vi "Move Main VI Controls.vi"(8 "error in":errorcluster, 11 "VIRef in":refnum<vi>) -> (0 "error out":errorcluster)   [LabVIEW 2018]
uses:
  <vilib>/Utility/miscctls.llb/LVPointTypeDef.ctl
panel:
  out "Height":i16
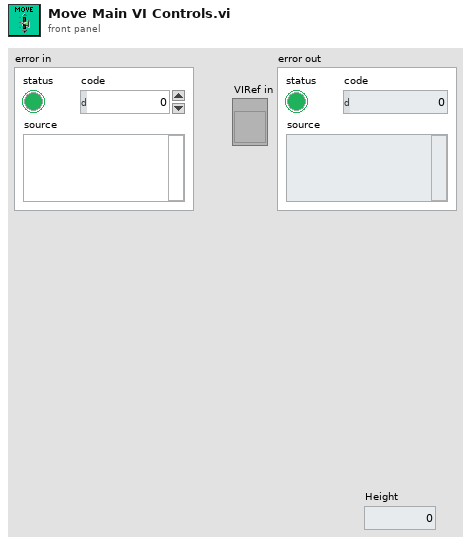
[diagram p1: front panel]
types:
  T1 = typedef "LVPointTypeDef.ctl" = cluster{"Horizontal":i16, "Vertical":i16}
  T2 = typedef "LVRectTypeDef.ctl" = cluster{"Left":i16, "Top":i16, "Right":i16, "Bottom":i16}
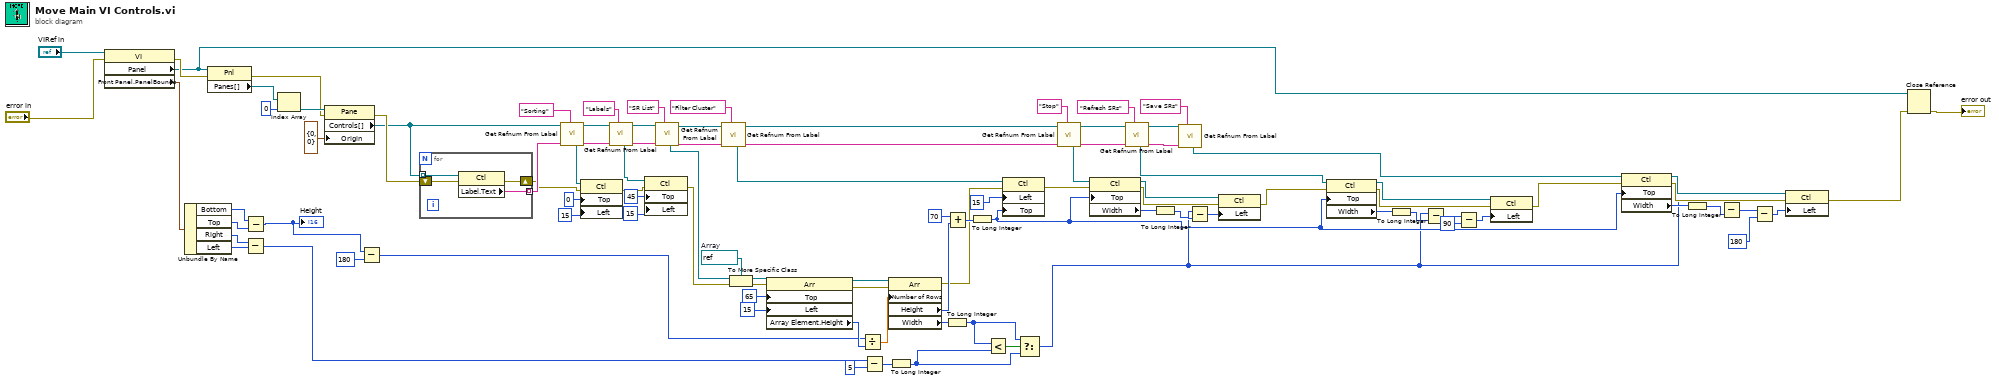
[diagram p0: block diagram]
diagram:
  w66 = refnum<vi> refnum  # Array
  n1 = property class="VI"(reference="VIRef in", error in="error in") -> (error out=w95:errorcluster, "Panel"=w3:refnum<vi>, "Front Panel.PanelBounds"=w92:T2)  [unwired: 1 out]
  n2 = Unbundle By Name(w92) -> ("Bottom"=w52:i16, "Top"=w51:i16, "Right"=w42:i16, "Left"=w41:i16)
  n3 = property class="Pnl"(reference=w3, error in=w95) -> (error out=w94:errorcluster, "Panes[]"=w96:refnum<vi>[])  [unwired: 1 out]
  n4 = Subtract(x=w42, y=w41) -> (x-y=w13:i16)
  n5 = Subtract(x=w52, y=w51) -> (x-y=w49:i16)
  "Height" <- w49
  n6 = Index Array(array=w96, index=0) -> (element=w97:refnum<vi>)
  n7 = property class="Pane"(reference=w97, error in=w94, "Origin"=T1 {"Horizontal"=0, "Vertical"=0}) -> (error out=w93:errorcluster, "Controls[]"=w90:refnum<vi>[])  [unwired: 1 out]
  n8 = Subtract(x=w49, y=i16 180) -> (x-y=w48:i16)
  n9 = for {
    tunnel: w90 -> [w102] mode=indexing
    shift-right: [w103] -> w58
    shift-left: w93 -> [w104]
    tunnel: [w101] -> w89 mode=indexing
    n10 = property class="Ctl"(reference=w102, error in=w104) -> (error out=w103:errorcluster, "Label.Text"=w101:string)  [unwired: 1 out]
  }
  n11 = call "Get Refnum From Label.vi"("label"="Sorting" ("element"), "label array in"=w89, "controls[] in"=w90) -> ("label array out"=w86:string[], "controls[] out"=w87:refnum<vi>[], "refnum out"=w70:refnum<vi>)  [unwired: 6 in]
  n12 = property class="Ctl"(reference=w70, error in=w58, "Top"=0 ("Position:Left"), "Left"=15 ("Position:Top")) -> (error out=w61:errorcluster)  [unwired: 1 out]
  n13 = call "Get Refnum From Label.vi"("label"="Labels" ("element"), "label array in"=w86, "controls[] in"=w87) -> ("label array out"=w83:string[], "controls[] out"=w84:refnum<vi>[], "refnum out"=w69:refnum<vi>)  [unwired: 6 in]
  n14 = property class="Ctl"(reference=w69, error in=w61, "Top"=45 ("Position:Top"), "Left"=15 ("Position:Left")) -> (error out=w60:errorcluster)  [unwired: 1 out]
  n15 = call "Get Refnum From Label.vi"("label"="SR List" ("element"), "label array in"=w83, "controls[] in"=w84) -> ("label array out"=w85:string[], "controls[] out"=w82:refnum<vi>[], "refnum out"=w67:refnum<vi>)  [unwired: 6 in]
  n16 = call "Get Refnum From Label.vi"("label"="Filter Cluster" ("element"), "label array in"=w85, "controls[] in"=w82) -> ("label array out"=w77:string[], "controls[] out"=w78:refnum<vi>[], "refnum out"=w47:refnum<vi>)  [unwired: 6 in]
  n17 = To More Specific Class(target class=w66, reference=w67, error in=w60) -> (specific class reference=w62:refnum<vi>, error out=w59:errorcluster)
  n18 = property class="Arr"(reference=w62, error in=w59, "Top"=65 ("Position:Top"), "Left"=15 ("Position:Left")) -> (reference out=w56:refnum<vi>, error out=w55:errorcluster, "Array Element.Height"=w54:u32)
  n19 = Divide(x=w48, y=w54) -> (x/y=w53:dbl)
  n20 = Subtract(x=w13, y=i16 5) -> (x-y=w10:i16)
  n21 = property class="Arr"(reference=w56, error in=w55, "Number of Rows"=w53) -> (error out=w40:errorcluster, "Height"=w45:u32, "Width"=w11:u32)  [unwired: 1 out]
  n22 = To Long Integer(number=w10) -> (32bit integer=w7:i32)
  n23 = To Long Integer(number=w11) -> (32bit integer=w8:i32)
  n24 = Add(x=u32 70, y=w45) -> (x+y=w43:u32)
  n25 = To Long Integer(number=w43) -> (32bit integer=w17:i32)
  n26 = Less?(x=w8, y=w7) -> (x < y?=w9:bool)
  n27 = property class="Ctl"(reference=w47, error in=w40, "Left"=15 ("Position:Left"), "Top"=w17) -> (error out=w5:errorcluster)  [unwired: 1 out]
  n28 = Select(t=w8, s=w9, f=w7) -> (s? t:f=w6:i32)
  n29 = call "Get Refnum From Label.vi"("label"="Stop" ("element"), "label array in"=w77, "controls[] in"=w78) -> ("label array out"=w71:string[], "controls[] out"=w74:refnum<vi>[], "refnum out"=w38:refnum<vi>)  [unwired: 6 in]
  n30 = property class="Ctl"(reference=w38, error in=w5, "Top"=w17) -> (reference out=w35:refnum<vi>, error out=w34:errorcluster, "Width"=w36:u32)
  n31 = call "Get Refnum From Label.vi"("label"="Refresh SRs" ("element"), "label array in"=w71, "controls[] in"=w74) -> ("label array out"=w72:string[], "controls[] out"=w73:refnum<vi>[], "refnum out"=w30:refnum<vi>)  [unwired: 6 in]
  n32 = To Long Integer(number=w36) -> (32bit integer=w16:i32)
  n33 = call "Get Refnum From Label.vi"("label"="Save SRs" ("element"), "label array in"=w72, "controls[] in"=w73) -> ("refnum out"=w20:refnum<vi>)  [unwired: 6 in, 2 out]
  n34 = Subtract(x=w6, y=w16) -> (x-y=w37:i32)
  n35 = property class="Ctl"(reference=w35, error in=w34, "Left"=w37) -> (error out=w19:errorcluster)  [unwired: 1 out]
  n36 = property class="Ctl"(reference=w30, error in=w19, "Top"=w17) -> (reference out=w32:refnum<vi>, error out=w33:errorcluster, "Width"=w31:u32)
  n37 = To Long Integer(number=w31) -> (32bit integer=w15:i32)
  n38 = Subtract(x=w6, y=w15) -> (x-y=w29:i32)
  n39 = Subtract(x=w29, y=90) -> (x-y=w27:i32)
  n40 = property class="Ctl"(reference=w32, error in=w33, "Left"=w27) -> (error out=w18:errorcluster)  [unwired: 1 out]
  n41 = property class="Ctl"(reference=w20, error in=w18, "Top"=w17) -> (reference out=w22:refnum<vi>, error out=w21:errorcluster, "Width"=w23:u32)
  n42 = To Long Integer(number=w23) -> (32bit integer=w14:i32)
  n43 = Subtract(x=w6, y=w14) -> (x-y=w24:i32)
  n44 = Subtract(x=w24, y=180) -> (x-y=w26:i32)
  n45 = property class="Ctl"(reference=w22, error in=w21, "Left"=w26) -> (error out=w4:errorcluster)  [unwired: 1 out]
  n46 = Close Reference(reference=w3, error in (no error)=w4) -> (error out=→"error out":errorcluster)
